vi "vipcApply.vi"() -> ()   [LabVIEW 2014, in "lv-cli-steps.lvlib"]
uses:
  lv-cli-steps.lvlib
  <vilib>/Utility/error.llb/DialogType.ctl
  <vilib>/Wiresmith Technology/LabVIEW CLI/CLI Class/CLI.lvclass
  <vilib>/JKI/VIPM API/VIPM API_vipm_api.lvlib
panel:
  out "error out":errorcluster
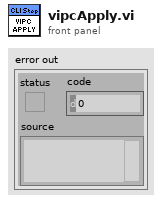
[diagram p1: front panel]
types:
  T1 = typedef "DialogType.ctl" = u16
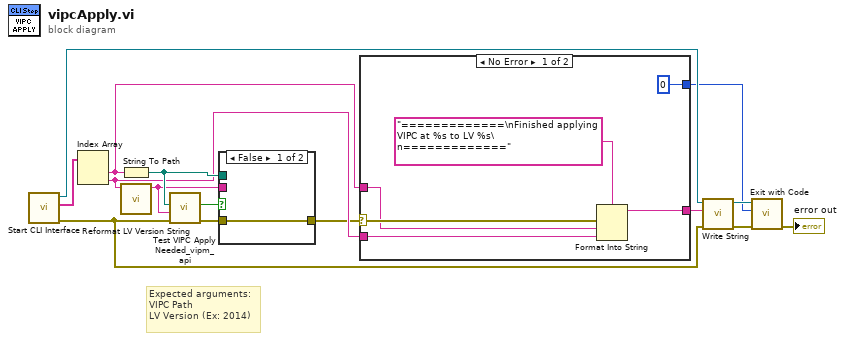
[diagram p0: block diagram]
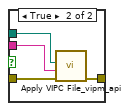
[diagram p2: hidden frame]
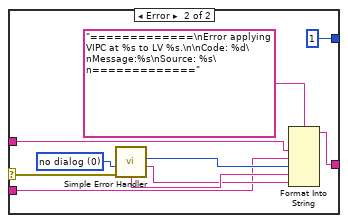
[diagram p3: hidden frame]
diagram:
  # "Expected arguments:\nVIPC Path\nLV Version (Ex: 2014)"
  n1 = call <vilib>:"Start CLI Interface.vi"() -> ("error out"=w1:errorcluster, "Custom Parameters"=w15:string[], "CLI out"=w13:refnum<class "CLI.lvclass">)  [unwired: 9 in]
  n2 = Index Array(array=w15) -> (element #1=w6:string, element #2=w4:string)  [unwired: 2 in]
  n3 = String To Path(string=w6) -> (path=w5:path)
  n4 = call "Reformat LV Version String.vi"("Version String (2014)"=w4) -> ("Short Version String (14.0)"=w3:string)  [unwired: 10 in]
  n5 = call <vilib>:"Test VIPC Apply Needed_vipm_api.vi"("error in (no error)"=w1, "LabVIEW Version (use vipc version)"=w3, "VIPC File Path"=w5) -> ("error out"=w8:errorcluster, "Need to Apply?"=w7:bool)  [unwired: 7 in]
  n6 = case shown="False" w7 {
    tunnel: w8 -> [w16 w20]
    tunnel: w5 -> [_ w19]
    tunnel: w3 -> [_ w18]
    tunnel: [w16 w17] -> w2
    frame False {
    }
    frame True {
      n7 = call <vilib>:"Apply VIPC File_vipm_api.vi"("error in (no error)"=w20, "LabVIEW Version"=w18, "VIPC File"=w19) -> ("error out"=w17:errorcluster)  [unwired: 8 in]
    }
  }
  n8 = case shown="No Error" w2 {
    selector: w2 -> [w25 w35]
    tunnel: w6 -> [w24 w31]
    tunnel: [w23 w36] -> w14
    tunnel: [0 ("Exit Code (0)") 1 ("Exit Code (0)")] -> w10
    tunnel: w4 -> [w21 w27]
    frame No Error {
      n9 = Format Into String(format string="=============\nFinished applying VIPC at %s to LV %s\n=============", error in=w25, w24, w21) -> (resulting string=w23:string)  [unwired: 1 in, 1 out]
    }
    frame Error {
      w34 = T1 0 items=["no dialog", "OK message", "continue or stop message", "OK message + warnings", "continue/stop + warnings"] ("type of dialog (OK msg:1)")
      n10 = call <vilib>:"Simple Error Handler.vi"("type of dialog (OK msg:1)"=w34, "error in (no error)"=w35) -> ("code out"=w28:i32, "source out"=w29:string, "message"=w30:string)  [unwired: 3 in, 2 out]
      n11 = Format Into String(format string="=============\nError applying VIPC at %s to LV %s.\n\nCode: %d\nMessage:%s\nSource: %s\n=============", w31, w27, w28, w30, w29) -> (resulting string=w36:string)  [unwired: 2 in, 1 out]
    }
  }
  n12 = call <vilib>:"Write String.vi"("error in (no error)"=w1, "Text to Write"=w14, "CLI in"=w13) -> ("error out"=w12:errorcluster, "CLI out"=w11:refnum<class "CLI.lvclass">)  [unwired: 7 in]
  n13 = call <vilib>:"Exit with Code.vi"("error in (no error)"=w12, "Exit Code (0)"=w10, "CLI in"=w11) -> ("error out"=→"error out":errorcluster)  [unwired: 8 in]
